vi "Finish.vi"(8 "error in (no error)":errorcluster, 11 "EventMgr in":refnum<class "EventMgr.lvclass">) -> (0 "error out":errorcluster, 3 "EventMgr out":refnum<class "EventMgr.lvclass">)   [LabVIEW 2013, in "EventMgr.lvclass"]
uses:
  EventMgr.lvclass
  System/System.lvclass
  EventMgr.lvclass/EventMgr.ctl
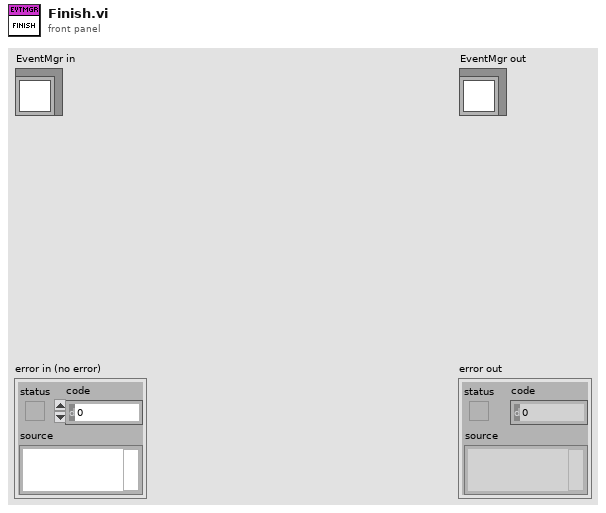
[diagram p1: front panel]
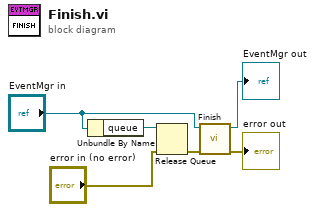
[diagram p0: block diagram]
diagram:
  n1 = Unbundle By Name("EventMgr in") -> ("queue"=w3:refnum<queue>)
  n2 = Release Queue(queue=w3, error in (no error)="error in (no error)") -> (error out=w1:errorcluster)  [unwired: 1 in, 2 out]
  n3 = call-parent "Finish.vi"("error in (no error)"=w1, "System in"="EventMgr in") -> ("error out"=→"error out":errorcluster, "System out"=→"EventMgr out":refnum<class "EventMgr.lvclass">)  [unwired: 8 in]
